vi "Act Tabla.vi"(8 "error in (no error)":errorcluster, 11 "Nestle  Actor in":refnum<class "Nestle  Actor.lvclass">) -> (0 "error out":errorcluster, 3 "Nestle  Actor out":refnum<class "Nestle  Actor.lvclass">)   [LabVIEW 2020, in "Nestle  Actor.lvlib" / "Nestle  Actor.lvclass"]
uses:
  Nestle  Actor.lvclass
  Nestle  Actor.lvclass/Nestle  Actor.ctl
  <vilib>/Utility/config.llb/Read Key (Double).vi
  <vilib>/Utility/config.llb/NI_LVConfig.lvlib
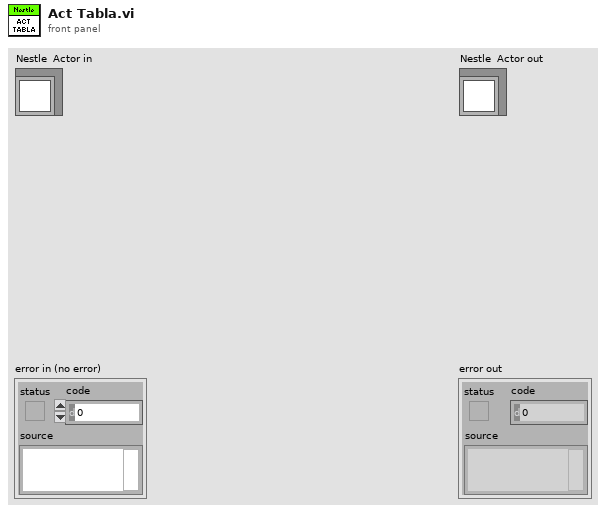
[diagram p1: front panel]
types:
  T1 = typedef "NI_LVConfig.lvlib/Config Data RefNum.ctl" = refnum<k1>
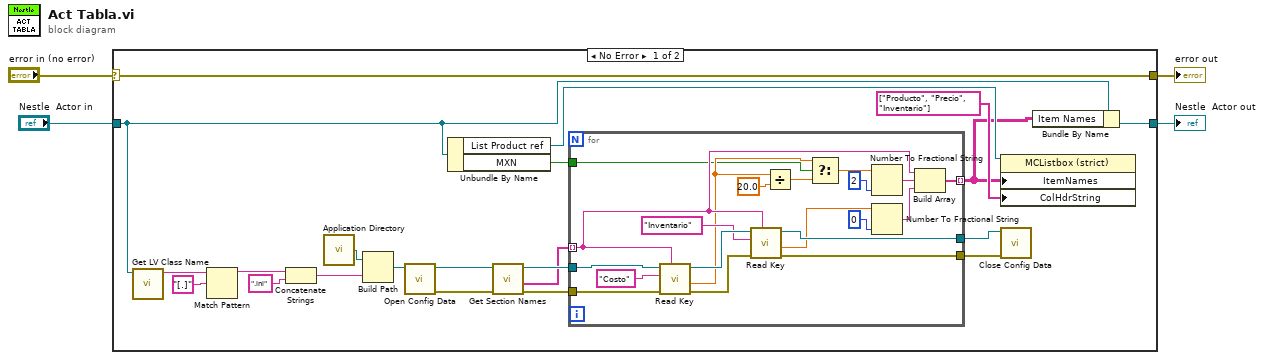
[diagram p0: block diagram]
diagram:
  n1 = case shown="No Error" "error in (no error)" {
    selector: "error in (no error)" -> [w25 w47]
    tunnel: [w25 w47] -> w3
    tunnel: [w6 w46] -> w1
    tunnel: "Nestle  Actor in" -> [w7 w46]
    frame No Error {
      n2 = call <vilib>:"Get LV Class Name.vi"("object"=w7) -> ("class name"=w18:string)  [unwired: 9 in, 1 out]
      n3 = Match Pattern(string=w18, regular expression="[.]") -> (before substring=w17:string)  [unwired: 1 in, 3 out]
      n4 = Concatenate Strings(w17, ".ini" ("string")) -> (w24:string)
      n5 = call <vilib>:"Application Directory.vi"() -> ("Application Directory"=w22:path)
      n6 = Build Path(base path=w22, name or relative path=w24) -> (appended path=w21:path)
      n7 = call <vilib>:"Open Config Data.vi"("configuration file path"=w21) -> ("error out"=w14:errorcluster, "refnum"=w15:T1)  [unwired: 8 in, 1 out]
      n8 = Unbundle By Name(w7) -> ("List Product ref"=w8:refnum<vi>, "MXN"=w10:bool)
      n9 = call <vilib>:"Get Section Names.vi"("error in (no error)"=w14, "refnum"=w15) -> ("error out"=w12:errorcluster, "section names"=w11:string[], "refnum out"=w13:T1)  [unwired: 7 in]
      n10 = for {
        tunnel: w13 -> [w45]
        tunnel: [w42] -> w20
        tunnel: [w41] -> w19
        tunnel: w12 -> [w38]
        tunnel: w11 -> [w37] mode=indexing
        tunnel: w10 -> [w26]
        tunnel: [w36] -> w5 mode=indexing
        n11 = call-poly <vilib>:"Read Key.vi"("section"=w37, "error in (no error)"=w38, "key"="Costo", "refnum"=w45) -> ("error out"=w44:errorcluster, "value"=w32:dbl, "refnum out"=w43:T1)  [unwired: 4 in, 1 out]
        n12 = call-poly <vilib>:"Read Key.vi"("section"=w37, "error in (no error)"=w44, "key"="Inventario", "refnum"=w43) -> ("error out"=w41:errorcluster, "value"=w30:dbl, "refnum out"=w42:T1)  [unwired: 4 in, 1 out]
        n13 = Divide(x=w32, y=20.0) -> (x/y=w34:dbl)
        n14 = Select(t=w32, s=w26, f=w34) -> (s? t:f=w33:dbl)
        n15 = Number To Fractional String(number=w33, precision (6)=i16 2) -> (F-format string=w27:string)  [unwired: 2 in]
        n16 = Number To Fractional String(number=w30, precision (6)=i16 0) -> (F-format string=w28:string)  [unwired: 2 in]
        n17 = Build Array(w37, w27, w28) -> (w36:string[])
      }
      n18 = property class="MCListbox (strict)"(reference=w8, "ItemNames"=w5, "ColHdrString"=string[] ["Producto", "Precio", "Inventario"] ("Column Header Strings[]")) -> ()  [unwired: 1 in, 2 out]
      n19 = call <vilib>:"Close Config Data.vi"("error in (no error)"=w19, "refnum"=w20) -> ()  [unwired: 8 in, 2 out]
      n20 = Bundle By Name(cluster=w7, "Item Names"=w5) -> (w6:refnum<class "Nestle  Actor.lvclass">)
    }
    frame Error {
    }
  }
  "error out" <- w3
  "Nestle  Actor out" <- w1
